vi "Initialize.vi"(8 "error in (no error)":errorcluster, 11 "reference in":refnum<class "NISync.lvclass">) -> (0 "error out":errorcluster, 3 "reference out":refnum<class "NISync.lvclass">)   [LabVIEW 2019, in "NISync.lvclass"]
doc: "Initializes module"
uses:
  NISync.lvclass
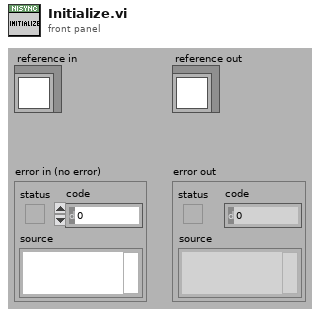
[diagram p1: front panel]
types:
  T1 = typedef "NISync.lvclass/ObjectAttributesRef.ctl" = refnum<data-value>
  T2 = typedef "NISync.lvclass/ObjectAttributes.ctl" = cluster{"Timing module":tag, "mode":enum16{"None", "Export trig", "Import trig"}, "Module terminal":string, "PXI line":string}
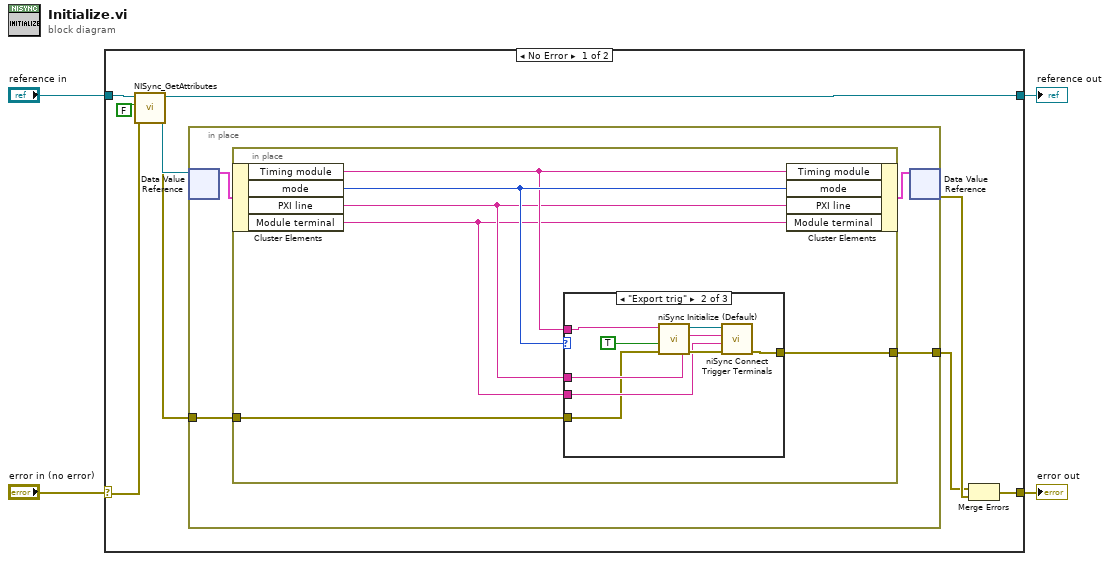
[diagram p0: block diagram]
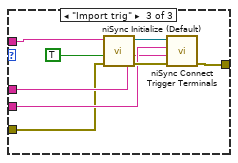
[diagram p3: hidden frame]
diagram:
  n1 = case shown="No Error" "error in (no error)" {
    selector: "error in (no error)" -> [w9 w42]
    tunnel: [w13 w42] -> w3
    tunnel: [w8 w41] -> w1
    tunnel: "reference in" -> [w11 w41]
    frame No Error {
      n2 = call "NISync_GetAttributes.vi"("error in (no error)"=w9, "return data? (T)"=FALSE, "reference in"=w11) -> ("error out"=w6:errorcluster, "attributes ref"=w7:T1, "reference out"=w8:refnum<class "NISync.lvclass">)  [unwired: 5 in, 1 out]
      n3 = in-place {
        in-place-border: w6 -> [w15]
        in-place-border: [w14] -> w5
        n4 = in-place-dvr #1(w7) -> (w16:T2)  [unwired: 1 out]
        n5 = in-place {
          in-place-border: w15 -> [w23]
          in-place-border: [w18] -> w14
          n6 = in-place-cluster #2(w16) -> ("Timing module"=w21:tag, "mode"=w22:enum16{"None", "Export trig", "Import trig"}, "PXI line"=w20:string, "Module terminal"=w19:string)
          n7 = case shown="\"Export trig\"" w22 {
            tunnel: w21 -> [_ w29 w37]
            tunnel: [w24 w28 w36] -> w18
            tunnel: w20 -> [_ w27 w34]
            tunnel: w19 -> [_ w26 w35]
            tunnel: w23 -> [w24 w25 w33]
            frame "None", Default {
            }
            frame "Export trig" {
              n8 = call <instrlib>:"niSync Initialize (Default).vi"("error in (no error)"=w25, "reset device (F)"=TRUE ("reset device (False)"), "resource name"=w29) -> ("error out"=w32:errorcluster, "instrument handle out"=w31:refnum<k15>)  [unwired: 7 in]
              n9 = call <instrlib>:"niSync Connect Trigger Terminals.vi"("error in (no error)"=w32, "destination terminal"=w26, "source terminal"=w27, "instrument handle"=w31) -> ("error out"=w28:errorcluster)  [unwired: 6 in, 1 out]
            }
            frame "Import trig" {
              n10 = call <instrlib>:"niSync Initialize (Default).vi"("error in (no error)"=w33, "reset device (F)"=TRUE ("reset device (False)"), "resource name"=w37) -> ("error out"=w40:errorcluster, "instrument handle out"=w39:refnum<k15>)  [unwired: 7 in]
              n11 = call <instrlib>:"niSync Connect Trigger Terminals.vi"("error in (no error)"=w40, "destination terminal"=w34, "source terminal"=w35, "instrument handle"=w39) -> ("error out"=w36:errorcluster)  [unwired: 6 in, 1 out]
            }
          }
          n12 = in-place-cluster #2("Timing module"=w21, "mode"=w22, "PXI line"=w20, "Module terminal"=w19) -> (w17:T2)
        }
        n13 = in-place-dvr #1(w17) -> (w12:errorcluster)  [unwired: 1 out]
      }
      n14 = Merge Errors(w5, w12) -> (w13:errorcluster)
    }
    frame Error {
    }
  }
  "error out" <- w3
  "reference out" <- w1
